vi "Write String.vi"(8 "error in (no error)":errorcluster, 11 "String":string) -> (0 "error out":errorcluster)   [LabVIEW 2015]
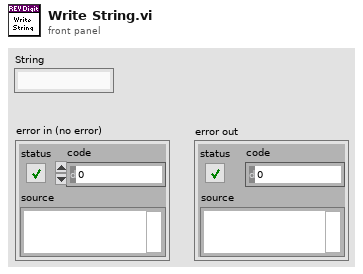
[diagram p1: front panel]
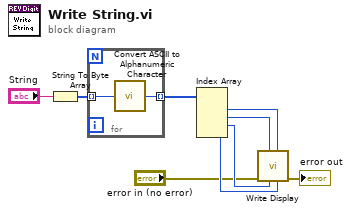
[diagram p0: block diagram]
diagram:
  n1 = String To Byte Array(string="String") -> (unsigned byte array=w1:u8[])
  n2 = for {
    tunnel: [w10] -> w7 mode=indexing
    tunnel: w1 -> [w11] mode=indexing
    n3 = call "Convert ASCII to Alphanumeric Character.vi"("ASCII Value"=w11) -> ("Alphanumeric Character Value"=w10:u16)
  }
  n4 = Index Array(array=w7) -> (element #1=w4:u16, element #2=w3:u16, element #3=w8:u16, element #4=w9:u16)  [unwired: 4 in]
  n5 = call "Write Display.vi"("D3"=w9, "D0"=w4, "D2"=w8, "D1"=w3, "error in (no error)"="error in (no error)") -> ("error out"=→"error out":errorcluster)  [unwired: 6 in]
